vi "FFT_0.2.vi"() -> ()   [LabVIEW 2011]
uses:
  <vilib>/Utility/file.llb/Read From Spreadsheet File (DBL).vi
  <vilib>/Analysis/2dsp.llb/Power Spectrum (DBL).vi
  <vilib>/Analysis/NI_AALPro.lvlib
panel:
  out "Freq Domain Signal 9":cluster{i32, dbl, "Power Spectrum":dbl[]}(graph)
  out "Frequency":dbl
  in  "sampl interval":dbl
  out "Freq Domain Signal 8":dbl[](graph)
  out "Time Domain Graph":waveform(dbl)(graph)
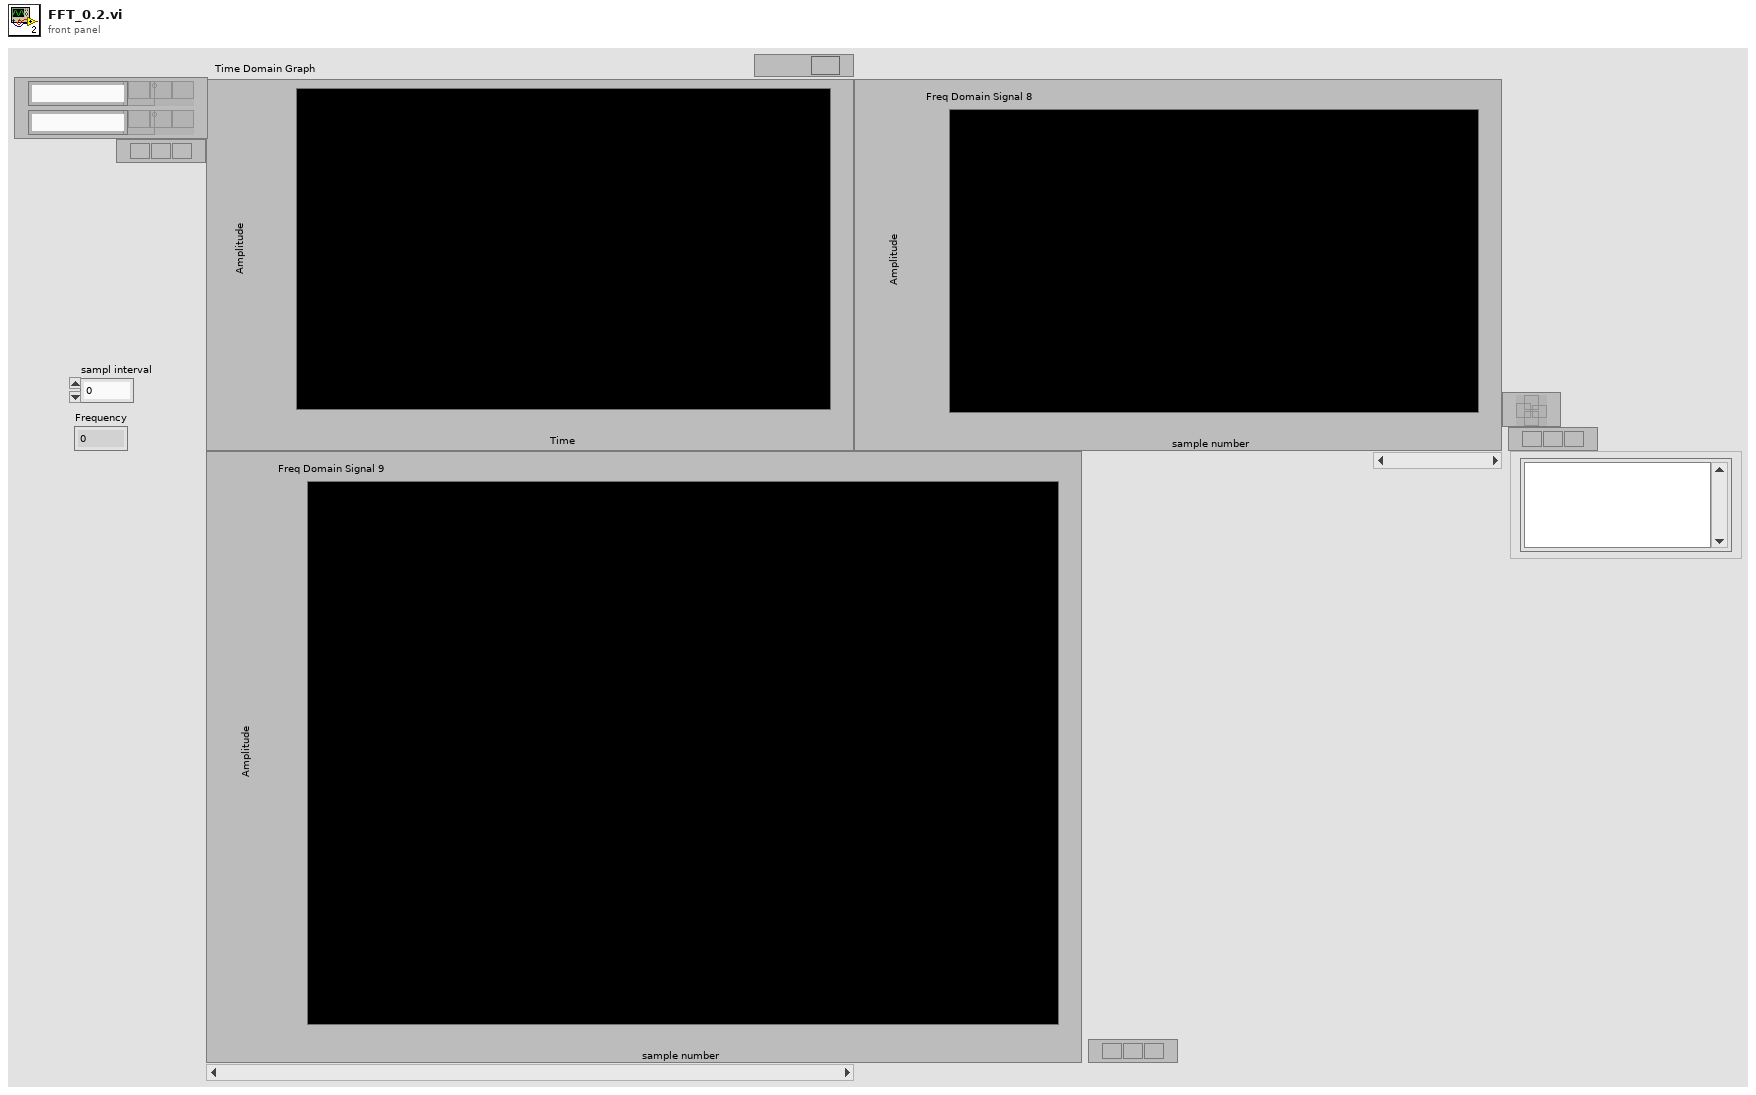
[diagram p1: front panel]
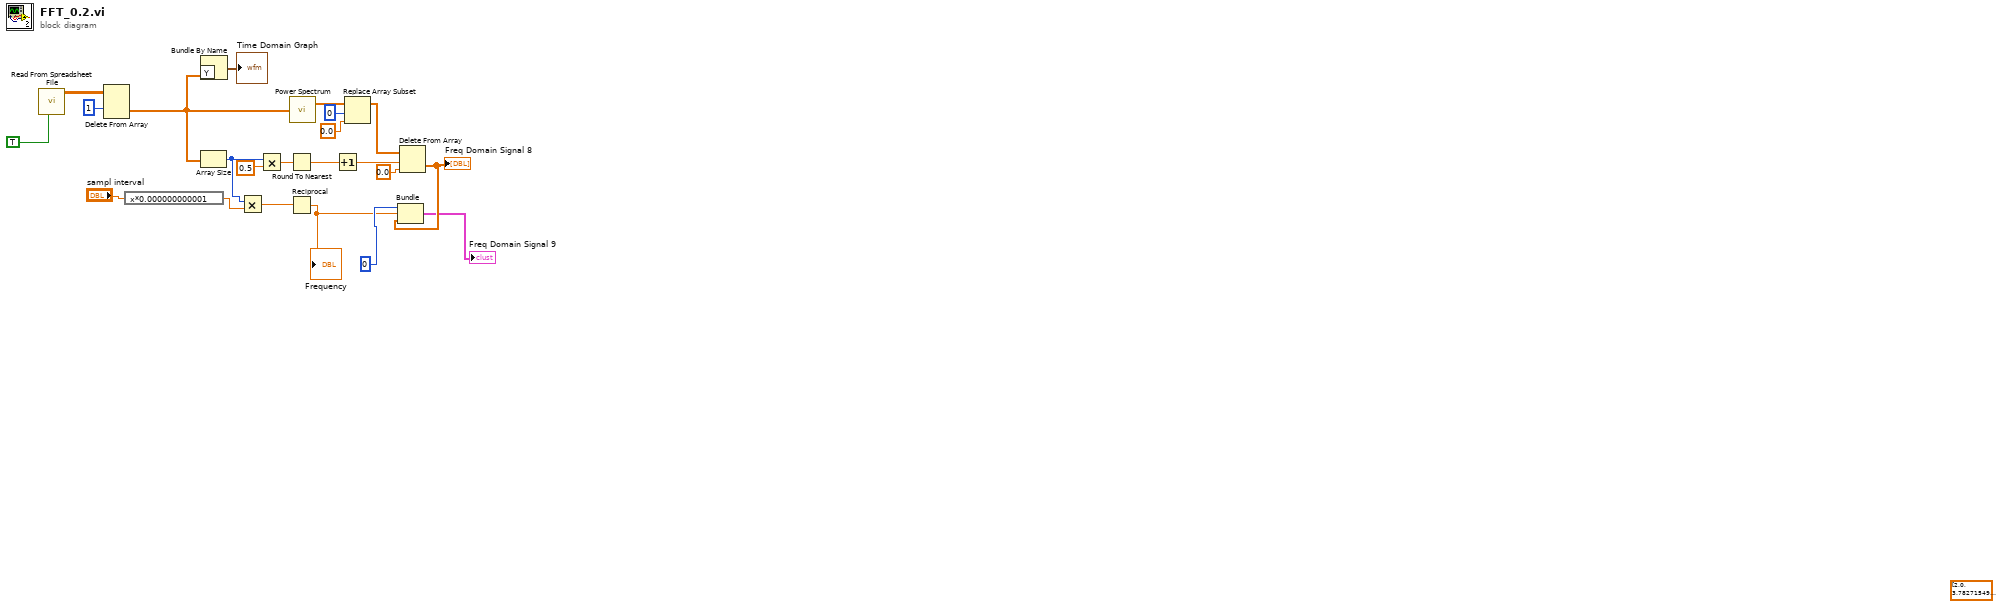
[diagram p0: block diagram]
diagram:
  (unwired) dbl[] [2.0, 3.782715492909256e-17, 2.3119858640185734e-17, 3.650732751486288e-17, 8.555768151167231e-17, 6.441967621258576e-17, 9.841929749359213e-17, 1.1330799082444038e-16, 1.123190351553056e-16, 1.1603236289277343e-16, 2.3375358987977577e-16, 1.487482793176421e-16, 1.9643330311990237e-16, 2.295516009326783e-16, 3.0850893123455297e-16, 3.861288231103786e-16, 5.60781734155656e-16, 6.21453523025715e-16, 1.0326766686211311e-15, 2.131328483980904e-15, 2.121320343559643, 2.1045038032792943e-15, 1.0232596243713128e-15, 7.538749575618319e-16, 5.175863178369834e-16, 4.789677440750349e-16, 4.3081654127118604e-16, 3.6241939367585564e-16, 3.376965885173409e-16, 2.905529767526317e-16, 2.3460231290928015e-16, 2.3775230472119654e-16, 2.3131233969930666e-16, 2.1278790042549664e-16, 2.450854665804215e-16, 1.8004359744274843e-16, 1.9117887898240092e-16, 1.6582490427410783e-16, 1.9090570075328726e-16, 1.4686208220082589e-16, 1.7448004707336706e-16, 1.4050870641224931e-16, 1.3353480736253179e-16, 1.1609193458109341e-16, 1.324988695828324e-16, 1.180384498324378e-16, 1.3212437174715926e-16, 1.321593619506191e-16, 1.1663338456383318e-16, 1.2494814803333557e-16, 4.7251312227837566e-17, 1.124563318019286e-16, 8.451006619467523e-17, 1.01834923263058e-16, 1.019748087258081e-16, 8.162169504592695e-17, 6.6890725156424e-17, 9.062603421497476e-17, 3.377154614691212e-17, 8.662967987276735e-17, 1.612402923888524e-16, 7.667630272857429e-17, 4.670649374334761e-17, 6.980592745364083e-17, 5.736062158104709e-17, 1.0179934274661244e-16, 6.910646334816405e-17, 6.524142973324831e-17, 6.589713036242515e-17, 5.240578100020998e-17, 1.4773771150638986e-16, 5.113004927797246e-17, 6.23023734432223e-17, 5.1637982820333345e-17, 5.693092357489852e-17, 6.884453663531953e-17, 8.104884936154391e-17, 3.2863449652773937e-17, 7.944835765365364e-17, 3.9239261584444213e-17, 2.223004752179044e-16, 2.736088165918919e-17, 7.75239459582e-17, 6.278867250568806e-17, 6.338104786289631e-17, 6.405106033117884e-17, 6.185071785361776e-17, 5.0221032702341656e-17, 7.22055294902605e-17, 5.712648877925192e-17, 1.5491023639103984e-16, 4.66779604582582e-17, 7.169628275505863e-17, 3.132320171315429e-17, 4.44337380137988e-17, 6.33386196683315e-17, 2.9507790850455154e-17, 3.288416480461804e-17, 1.6262058538107533e-17, 3.845754288702555e-17, 4.7251312227837566e-17, 4.5352878469721695e-17, 4.789871109292882e-17, 5.546786577257066e-17, 5.397572960363537e-17, 1.8190346320308198e-17, 4.5056277231329966e-17, 5.294736639703999e-17, 3.532836158279607e-17, 4.6425389349157565e-17, 9.323073243005851e-17, 3.8149881112680515e-17, 3.92432935567392e-17, 4.2463685427516037e-17, 6.207167417649316e-17, 4.020600398723522e-17, 7.26960944314611e-17, 4.454688592904438e-17, 6.629837927822503e-17, 4.16023611468932e-17, 2.2679951644582333e-16, 5.321835254886066e-17, 9.491780151010567e-17, 5.2367284072087276e-17, 9.425493406907125e-17, 7.674653053286961e-17, 7.212173768248606e-17, 4.874507423488851e-17, 6.615014796457917e-17, 5.1896375994449553e-17, 8.414539529746281e-17, 5.1796376909173514e-17, 8.069210677499387e-17, 5.231371848981001e-17, 7.990114259936454e-17, 2.146019984425651e-17, 6.400712755190212e-17, 4.0729098388609643e-17, 3.271104355493141e-17, 2.8735224948050246e-17, 1.5518216221891872e-16, 4.4408825170855186e-17, 2.7345292523300625e-17, 4.1793913257730446e-17, 4.529007307426247e-17, 8.094892566367416e-17, 5.1819722148675777e-17, 3.597211104412463e-17, 5.08322909327414e-17, 4.104073061956537e-17, 7.645422919767467e-17, 3.2561882973601364e-17, 2.4922120103521037e-17, 3.735322847794884e-17, 5.854433049481963e-18, 6.479536197298008e-17, 8.219175776477636e-18, 3.288731917788417e-17, 4.008049367669415e-17, 3.8195953546556795e-17, 1.2334137735869388e-16, 2.7179664217965278e-17, 3.518616243515674e-17, 4.122762009362606e-17, 4.9680933067185924e-17, 1.6070113352740578e-17, 5.525598122871273e-17, 3.626246066014676e-17, 4.313274463286765e-17, 3.5108682859998e-17, 2.80162094666575e-17, 1.7502219466658314e-17, 4.613060978389554e-17, 1.93858200182206e-17, 6.164588094618335e-17, 3.236751879052858e-17, 4.4145284354852904e-17, 2.7226258267151077e-17, 3.990035674680022e-17, 4.394094171771921e-17, 7.123602428212474e-17, 3.292943456880963e-17, 4.785339878816735e-17, 4.010190407778036e-17, 5.707620909122293e-17, 5.0508720938867234e-17, 5.978232943679899e-17, 4.22648566417199e-17, 5.035141292063648e-17, 2.3819509461181757e-17, 6.885389473271467e-17, 5.638420115759825e-18, 5.332218025159961e-18, 1.8334468036738116e-17, 1.5778093890281497e-17, 9.518588081324497e-18, 4.801375402208432e-17, 4.6713985631215024e-17, 3.32390389758952e-17, 7.546353313774506e-17, 7.645422919767467e-17, 3.8948988830632684e-17, 5.98563467489819e-17, 4.660494289242023e-17, 3.366197151108244e-17, 5.374839935934763e-17, 2.2488303094036495e-17, 2.4678323098033762e-17, 8.555011531259553e-18, 2.7463567382062714e-17, 3.798582301268292e-17, 3.361742055510472e-17, 4.0858239781303403e-17, 3.620466977547365e-17, 3.943315625131438e-17, 3.278696399196452e-17, 8.089623242768265e-17, 2.0789257287474012e-17, 3.605479945640452e-17, 3.733716880106881e-17, 9.314936733071274e-17, 2.37378962614456e-17, 2.1844966802028176e-17, 3.1129764357522416e-17, 2.1849003003822584e-17, 3.670625606673135e-17, 1.0563259020192478e-16, 4.770936710432679e-17, 8.783127288982596e-17, 2.5395410215754583e-17, 3.917352780915782e-16, 3.767348837505238e-17, 1.3057660322086161e-17, 5.554048750014832e-17, 5.603427297590493e-17, 6.159581718505446e-17, 4.5081115433475653e-17, 5.5175003858957385e-17, 2.712903978020735e-17, 8.279259520240502e-17, 1.8595019771327175e-18, 2.3466672817965984e-17, 1.262766115714541e-17, 6.512697278693294e-17, 5.2993671661334476e-17, 5.035725970683966e-17, 6.065317369441044e-17, 3.1776259461235776e-17, 2.8774447141554224e-17, 3.0385499480576006e-17] ("Freq Domain Signal 4")
  n1 = call-poly <vilib>:"Read From Spreadsheet File.vi"("transpose (no:F)"=TRUE) -> ("all rows"=w20:dbl[][])  [unwired: 6 in, 4 out]
  n2 = Delete From Array(array=w20, index (row)=1) -> (deleted portion=w15:dbl[])  [unwired: 2 in, 1 out]
  n3 = expression code="x*0.000000000001"("sampl interval") -> (w8:dbl)
  n4 = Bundle By Name("Y"=w15) -> (→"Time Domain Graph":waveform(dbl))  [unwired: 1 in]
  n5 = Array Size(array=w15) -> (size(s)=w7:i32)
  n6 = Multiply(x=w7, y=w8) -> (x*y=w6:dbl)
  n7 = Multiply(x=w7, y=0.5) -> (x*y=w17:dbl)
  n8 = Round To Nearest(number=w17) -> (nearest integer value=w16:dbl)
  n9 = Reciprocal(x=w6) -> (1/x=w4:dbl)
  "Frequency" <- w4
  n10 = call-poly <vilib>:"Power Spectrum.vi"("X"=w15) -> ("Power Spectrum"=w12:dbl[])  [unwired: 1 out]
  n11 = Increment(x=w16) -> (x+1=w10:dbl)
  n12 = Replace Array Subset(array=w12, new element=0.0 ("new element/subarray"), index=0) -> (w3:dbl[])
  n13 = Delete From Array(array=w3, length=w10, index=0.0 ("new element/subarray")) -> (deleted portion=w2:dbl[])  [unwired: 1 out]
  "Freq Domain Signal 8" <- w2
  n14 = Bundle(0, w4, "Power Spectrum"=w2) -> (→"Freq Domain Signal 9":cluster{i32, dbl, "Power Spectrum":dbl[]})  [unwired: 1 in]
